vi "Smooth.vi"(2 "Trigger":dbl, 3 "Yin":dbl, 4 "Xin":dbl) -> (0 "Y Output":dbl, 1 "X Output":dbl)   [LabVIEW 2016]
uses:
  <vilib>/Rock Robotics/Network Tables/NT Read Boolean.vi
  <vilib>/Rock Robotics/Network Tables/NT Read Number.vi
panel:
  in  "New Control?":bool
  out "yCurve":dbl
  out "x curve":dbl
  in  "Limits":cluster{dbl, dbl}(slide)={0.75, 0.5050505050505051} scale=0.0..1.0
  out "Yout from machine":dbl
  out "Xout from machine":dbl
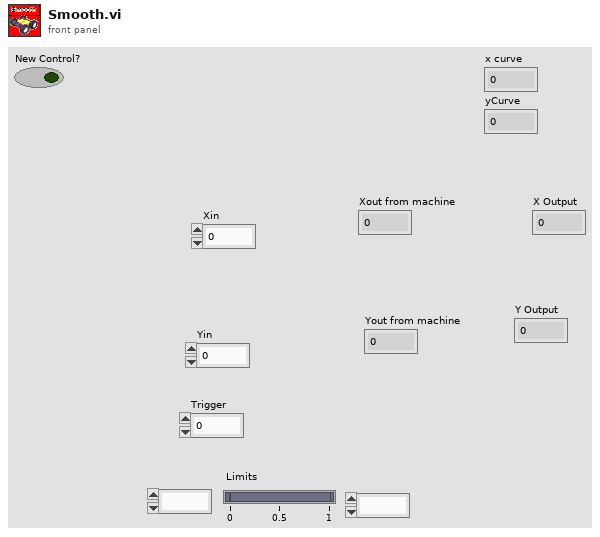
[diagram p1: front panel]
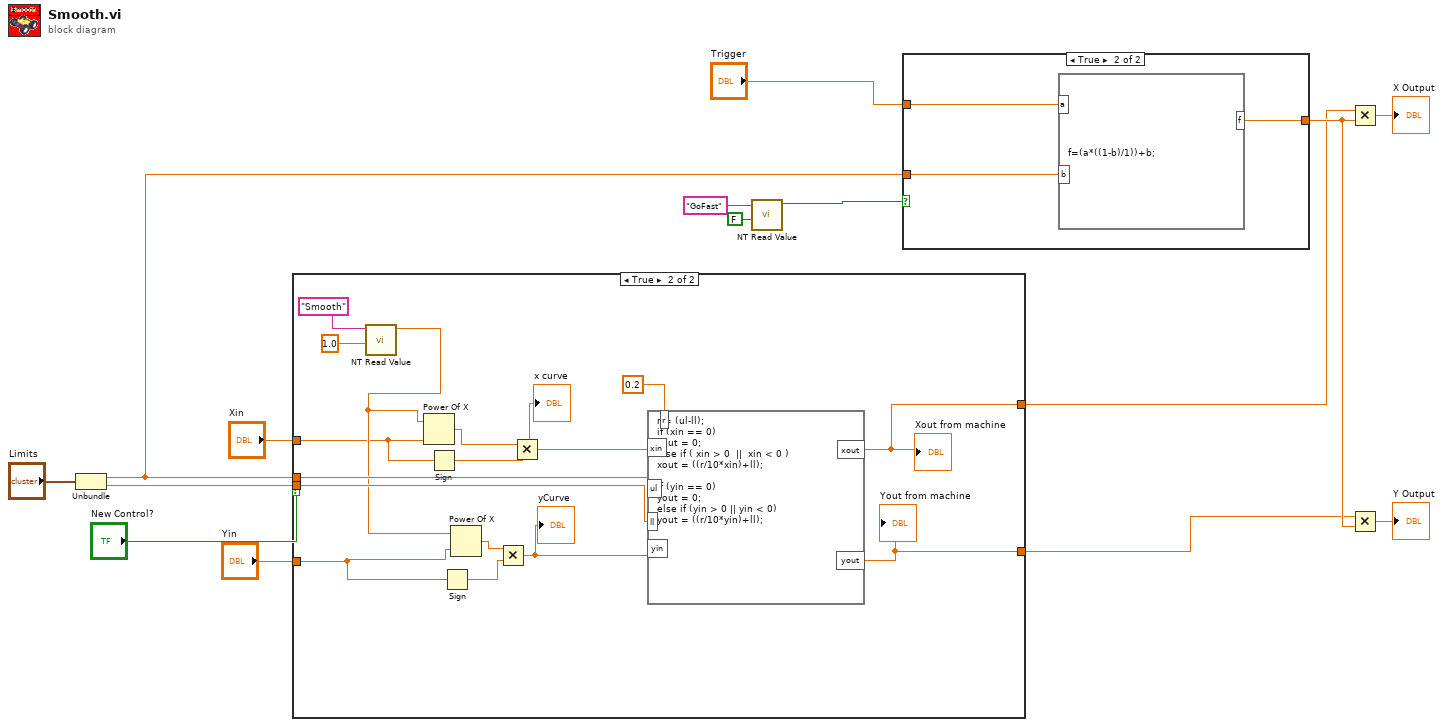
[diagram p0: block diagram]
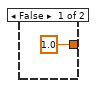
[diagram p3: hidden frame]
diagram:
  n1 = Unbundle("Limits") -> (w6:dbl, w7:dbl)
  n2 = case shown="True" "New Control?" {
    tunnel: w7 -> [_ w32]
    tunnel: w6 -> [_ w31]
    tunnel: [w17 w28] -> w5
    tunnel: [w16 w27] -> w4
    tunnel: "Xin" -> [w17 w19]
    tunnel: "Yin" -> [w16 w18]
    frame False {
    }
    frame True {
      n3 = call-poly <vilib>:"NT Read Value.vi"("Default Value"=1.0, "Name"="Smooth") -> ("Numeric"=w20:dbl)  [unwired: 8 in, 1 out]
      n4 = Power Of X(1:w19, 2:w20) -> (0:w25:dbl)
      n5 = Sign(1:w19) -> (0:w24:dbl)
      n6 = Sign(1:w18) -> (0:w26:dbl)
      n7 = Power Of X(1:w18, 2:w20) -> (0:w21:dbl)
      n8 = Multiply(x=w21, y=w26) -> (x*y=w22:dbl)
      "yCurve" <- w22
      n9 = Multiply(x=w25, y=w24) -> (x*y=w23:dbl)
      "x curve" <- w23
      n10 = formula code="r = (ul-ll);\nif (xin == 0)\nxout = 0;\nelse if ( xin > 0  ||  xin < 0 )\nxout = ((r/10*xin)+ll);\n\nif (yin == 0)\nyout = 0;\nelse if (yin > 0 || yin < 0)\nyout = ((r/10*yin)+ll);"("xin"=w23, "yin"=w22, "ul"=w31, "ll"=w32, "r"=0.2 ("input variable")) -> ("xout"=w28:dbl, "yout"=w27:dbl)
      "Xout from machine" <- w28
      "Yout from machine" <- w27
    }
  }
  n11 = call-poly <vilib>:"NT Read Value.vi"("Default Value"=FALSE, "Name"="GoFast") -> ("Boolean"=w13:bool)  [unwired: 8 in, 1 out]
  n12 = case shown="True" w13 {
    tunnel: [1.0 ("f") w35] -> w15
    tunnel: w6 -> [_ w36]
    tunnel: "Trigger" -> [_ w37]
    frame False {
    }
    frame True {
      n13 = formula code="f=(a*((1-b)/1))+b;"("a"=w37, "b"=w36) -> ("f"=w35:dbl)
    }
  }
  n14 = Multiply(x=w5, y=w15) -> (x*y=→"X Output":dbl)
  n15 = Multiply(x=w4, y=w15) -> (x*y=→"Y Output":dbl)
